vi "Get DDS Support Boxing Style.vi"(8 "error in (no error)":errorcluster, 11 "style":i32[](array[numeric])=[0, 0, 0, 0, 0, 0, 0, 0, 0, 0, 0, 0, 0, 0, 0, 0]) -> (0 "error out":errorcluster, 2 "function return":i32, 3 "style out":i32[](array[numeric]))   [LabVIEW 2021, in "vmmso.lvlib"]
doc: "DLL_API int WINAPI GetDDSSupportBoxingStyle(int* style);"
uses:
  vmmso.lvlib
  vmmso.dll
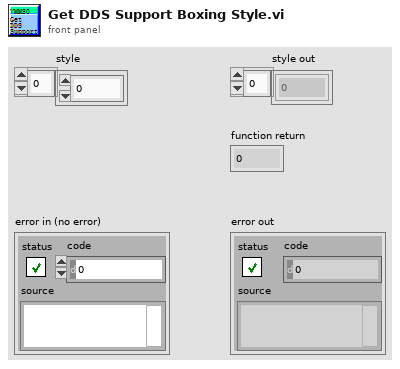
[diagram p1: front panel]
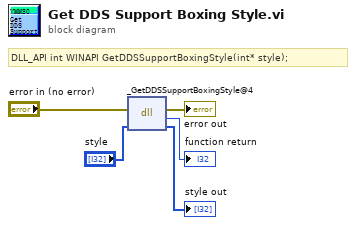
[diagram p0: block diagram]
diagram:
  # "DLL_API int WINAPI GetDDSSupportBoxingStyle(int* style);"
  n1 = dll-call lib="O:/MSO/library/demo-Labview/vmmso/vmmso.*" fn="_GetDDSSupportBoxingStyle@4"(error in="error in (no error)", "style"="style") -> (error out=→"error out":errorcluster, →"function return":i32, "style"=→"style out":i32[])  [unwired: 2 in, 1 out]
